vi "Configure Channel Characteristics.vi"(4 "Invert (F: Disable)":bool, 6 "Vernier (F: Disable)":bool, 8 "error in (no error)":errorcluster, 9 "BW Limit (F: Disable)":bool, 10 "Channel (1: Channel 1)":u16(ring)=1 items=["Channel 1"=1, "Channel 2"=2, "Channel 3"=3, "Channel 4"=4], 11 "VISA resource name":refnum<visa-resource-name>) -> (0 "error out":errorcluster, 3 "VISA resource name out":refnum<visa-resource-name>)   [LabVIEW 2023, in "RIGOL DS1054Z Driver.lvlib"]
doc: "Configure channel characteristics."
uses:
  <instrlib>/RIGOL-DS1054Z-LabVIEW/RIGOL DS1054Z Driver.lvlib
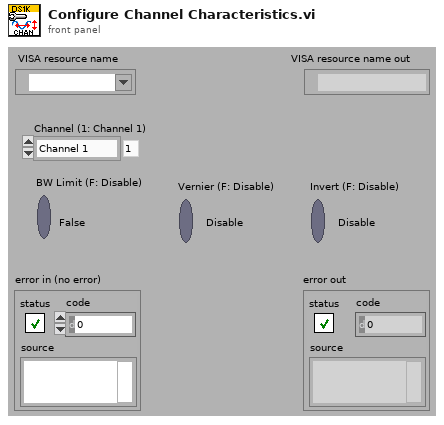
[diagram p1: front panel]
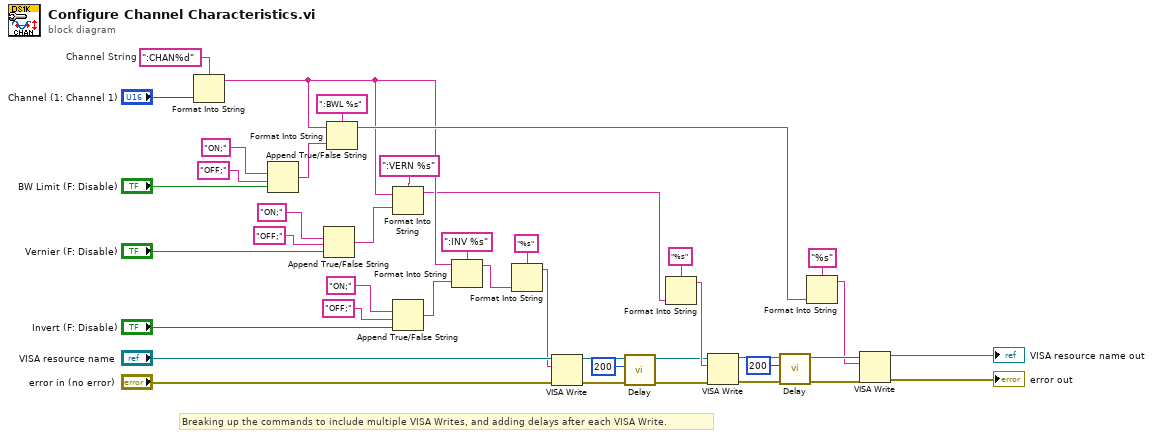
[diagram p0: block diagram]
diagram:
  w39 = ":CHAN%d"  # Channel String
  # "Breaking up the commands to include multiple VISA Writes, and adding delays after each VISA Write."
  n1 = Format Into String(format string=w39, "Channel (1: Channel 1)") -> (resulting string=w21:string)  [unwired: 2 in, 1 out]
  n2 = Append True/False String(1:"BW Limit (F: Disable)", 2:"OFF;" ("假字符串"), 3:"ON;" ("真字符串")) -> (0:w34:string)  [unwired: 1 out]
  n3 = Append True/False String(1:"Vernier (F: Disable)", 2:"OFF;" ("假字符串"), 3:"ON;" ("真字符串")) -> (0:w33:string)  [unwired: 1 out]
  n4 = Format Into String(format string=":BWL %s", initial string=w21, w34) -> (resulting string=w22:string)  [unwired: 1 in, 1 out]
  n5 = Format Into String(format string=":VERN %s", initial string=w21, w33) -> (resulting string=w18:string)  [unwired: 1 in, 1 out]
  n6 = Append True/False String(1:"Invert (F: Disable)", 2:"OFF;" ("假字符串"), 3:"ON;" ("真字符串")) -> (0:w28:string)  [unwired: 1 out]
  n7 = Format Into String(format string=":INV %s", initial string=w21, w28) -> (resulting string=w16:string)  [unwired: 1 in, 1 out]
  n8 = Format Into String(format string="%s", w16) -> (resulting string=w3:string)  [unwired: 2 in, 1 out]
  n9 = VISA Write(VISA resource name="VISA resource name", write buffer=w3, error in (no error)="error in (no error)") -> (VISA resource name out=w15:refnum<visa-resource-name>, error out=w14:errorcluster)  [unwired: 1 out]
  n10 = call <instrlib>:"Delay.vi"("error in (no error)"=w14, "Delay (ms)"=u32 200, "VISA resource name"=w15) -> ("error out"=w11:errorcluster, "VISA resource name out"=w12:refnum<visa-resource-name>)  [unwired: 7 out]
  n11 = Format Into String(format string="%s", w18) -> (resulting string=w13:string)  [unwired: 2 in, 1 out]
  n12 = VISA Write(VISA resource name=w12, write buffer=w13, error in (no error)=w11) -> (VISA resource name out=w10:refnum<visa-resource-name>, error out=w9:errorcluster)  [unwired: 1 out]
  n13 = call <instrlib>:"Delay.vi"("error in (no error)"=w9, "Delay (ms)"=u32 200, "VISA resource name"=w10) -> ("error out"=w7:errorcluster, "VISA resource name out"=w8:refnum<visa-resource-name>)  [unwired: 7 out]
  n14 = Format Into String(format string="%s", w22) -> (resulting string=w4:string)  [unwired: 2 in, 1 out]
  n15 = VISA Write(VISA resource name=w8, write buffer=w4, error in (no error)=w7) -> (VISA resource name out=→"VISA resource name out":refnum<visa-resource-name>, error out=→"error out":errorcluster)  [unwired: 1 out]
